vi "Sort LV Project Channels by Channel Index.vi"(8 "error in (no error)":errorcluster, 11 "Project Channels in":refnum<vi>[](array[refnum])) -> (0 "error out":errorcluster, 3 "Project Channels out":refnum<vi>[](array[refnum]))   [LabVIEW 2013, in "Scan Engine editor node.lvclass"]
uses:
  Scan Engine editor node.lvclass
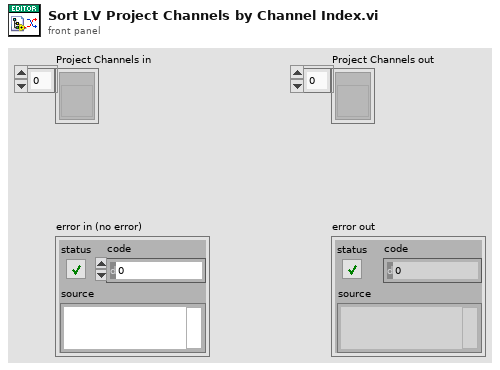
[diagram p1: front panel]
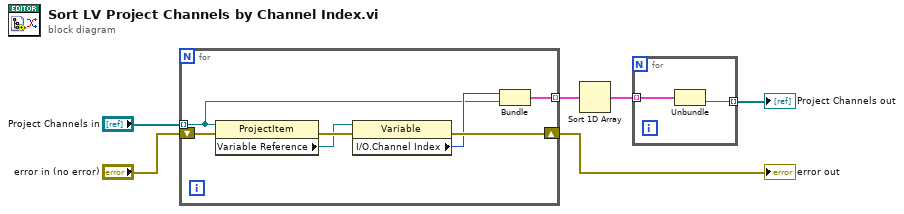
[diagram p0: block diagram]
diagram:
  n1 = for {
    tunnel: "Project Channels in" -> [w7] mode=indexing
    shift-right: [w13] -> w1
    shift-left: "error in (no error)" -> [w11]
    tunnel: [w9] -> w4 mode=indexing
    n2 = property class="ProjectItem"(reference=w7, error in=w11) -> (error out=w12:errorcluster, "Variable Reference"=w8:refnum<vi>)  [unwired: 1 out]
    n3 = property class="Variable"(reference=w8, error in=w12) -> (error out=w13:errorcluster, "I/O.Channel Index"=w10:u32)  [unwired: 1 out]
    n4 = Bundle("I/O.Channel Index"=w10, w7) -> (w9:cluster{"I/O.Channel Index":u32, refnum<vi>})  [unwired: 1 in]
  }
  "error out" <- w1
  n5 = Sort 1D Array(array=w4) -> (sorted array=w3:cluster{"I/O.Channel Index":u32, refnum<vi>}[])
  n6 = for {
    tunnel: w3 -> [w15] mode=indexing
    tunnel: [w14] -> w2 mode=indexing
    n7 = Unbundle(w15) -> (w14:refnum<vi>)  [unwired: 1 out]
  }
  "Project Channels out" <- w2
